vi "PS-RA03B FPGA.vi"() -> ()   [LabVIEW 2011]
uses:
  <vilib>/rvi/eio/common/nirviEmuTemplateMethod_errors.vi
  <vilib>/rvi/Memory/Memory_Emulation/niFpgaMemoryEmulationValidateCache.vi
  <vilib>/rvi/DataTransferAndStorage/Container/Common/niFpgaContainerGetUniqueNameForEmu.vi
  <vilib>/rvi/Memory/Memory_Emulation/nirvimemoryEmulationManagerCache_InsertValue.vi
  <vilib>/Utility/error.llb/Clear Errors.vi
  <vilib>/rvi/Memory/Memory_Emulation/nirvimemoryEmulationManagerCache_GetValue.vi
  <vilib>/rvi/Memory/Memory_Emulation/nirvimemoryEmulationManagerCache_SetValue.vi
  <vilib>/eio/EIONode/EIONode.xnode
  <vilib>/eio/EIOMethodNode/EIOMethodNode.xnode
  <vilib>/rvi/DataTransferAndStorage/Container/XNode/niFpgaContainer.xnode
  <vilib>/rvi/Memory/Memory_Emulation/nirvimemoryEmulation.vi
panel:
  out "Mod6/AO1":fxp<+/-,20,5> format="%.17g"
  out "Mod2/AO3":fxp<+/-,20,5> format="%.17g"
  out "Mod2/AO2":fxp<+/-,20,5> format="%.17g"
  out "Mod2/AO1":fxp<+/-,20,5> format="%.17g"
  out "Mod2/AO0":fxp<+/-,20,5> format="%.17g"
  out "Mod6/AO3":fxp<+/-,20,5> format="%.17g"
  out "Mod6/AO2":fxp<+/-,20,5> format="%.17g"
  out "Mod6/AO0":fxp<+/-,20,5> format="%.17g"
  out "Timestamp":u32 caption="Tick Count(Ticks)"
  out "Mod5/AI0":fxp<+/-,20,5> format="%.17g"
  out "Mod5/AI2":fxp<+/-,20,5> format="%.17g"
  out "Mod5/AI3":fxp<+/-,20,5> format="%.17g"
  out "Mod1/AI0":fxp<+/-,20,5> format="%.17g"
  out "Mod1/AI1":fxp<+/-,20,5> format="%.17g"
  out "Mod1/AI2":fxp<+/-,20,5> format="%.17g"
  out "Mod1/AI3":fxp<+/-,20,5> format="%.17g"
  out "Mod5/AI1":fxp<+/-,20,5> format="%.17g"
  out "period":u32
  out "delay":u32
  out "dperiod":u32
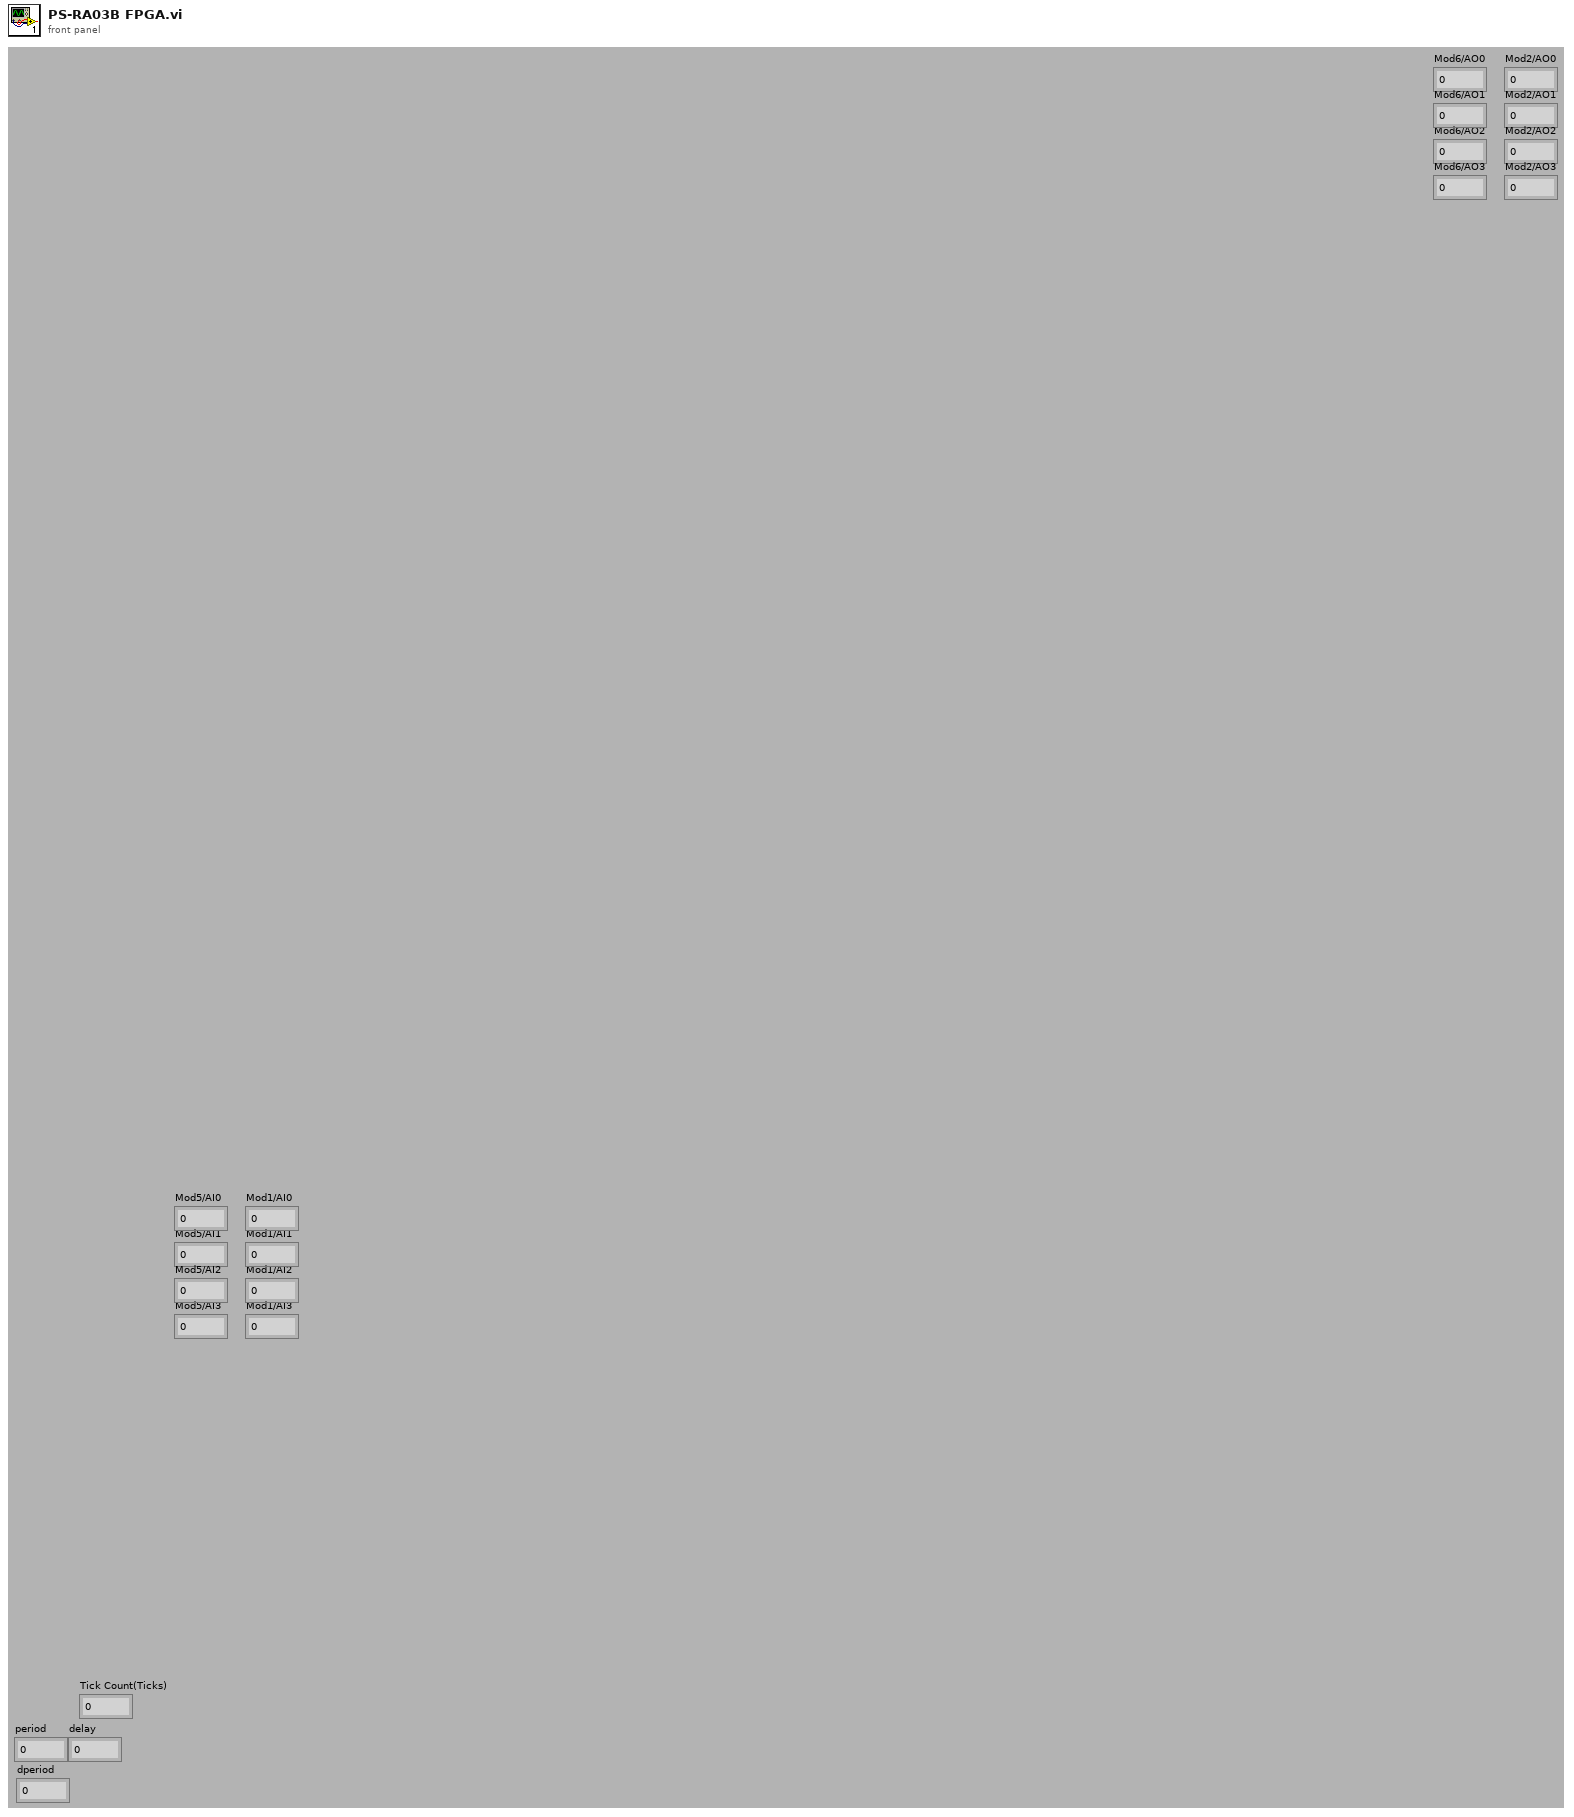
[diagram p1: front panel]
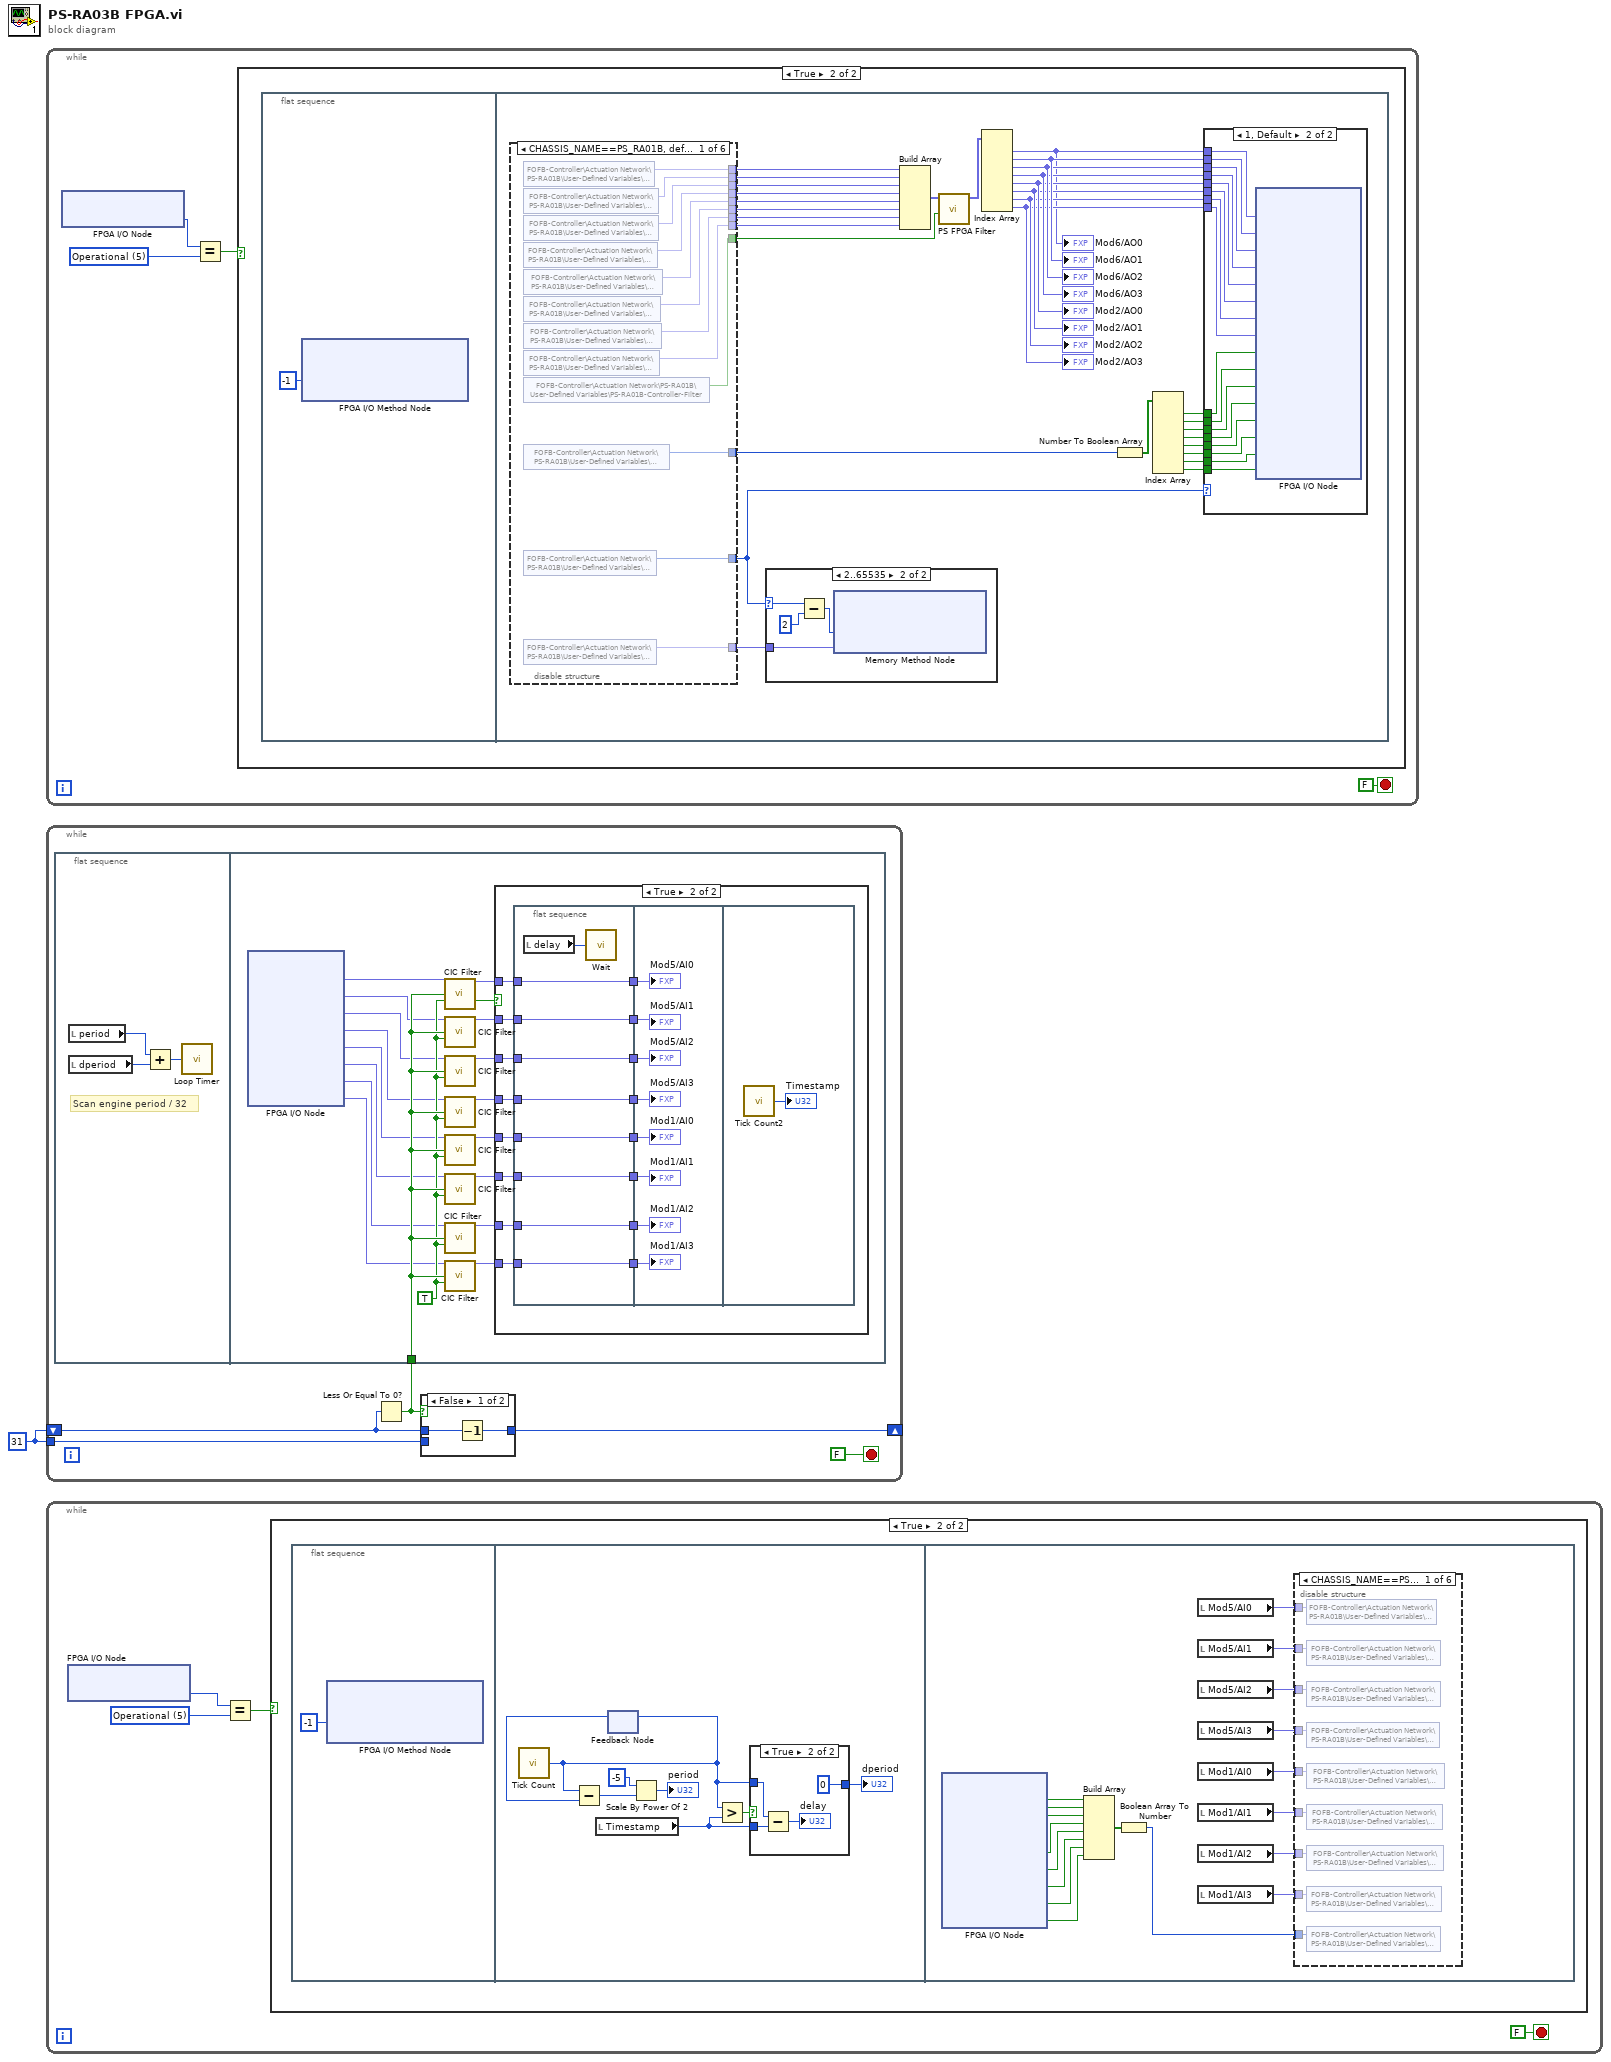
[diagram p0: block diagram]
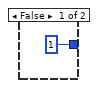
[diagram p5: hidden frame]
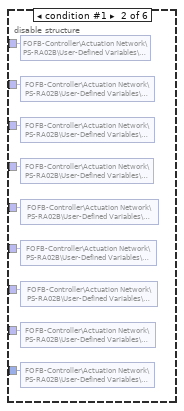
[diagram p6: hidden frame]
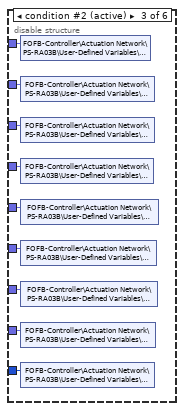
[diagram p7: hidden frame]
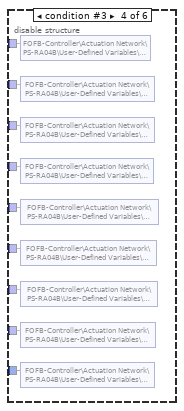
[diagram p8: hidden frame]
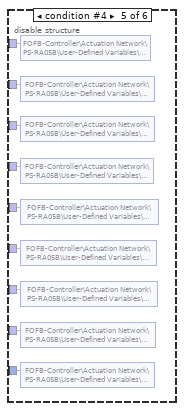
[diagram p9: hidden frame]
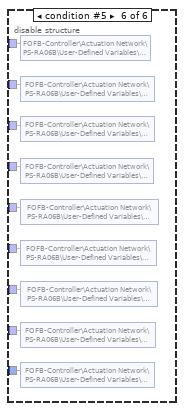
[diagram p10: hidden frame]
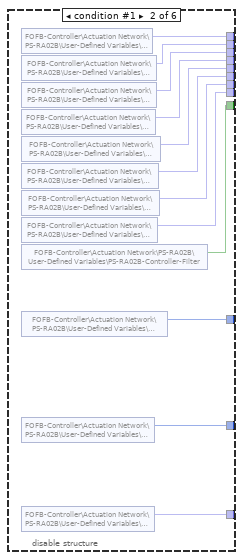
[diagram p14: hidden frame]
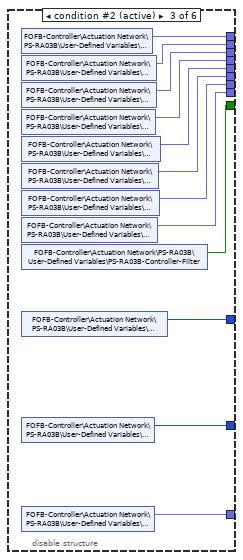
[diagram p15: hidden frame]
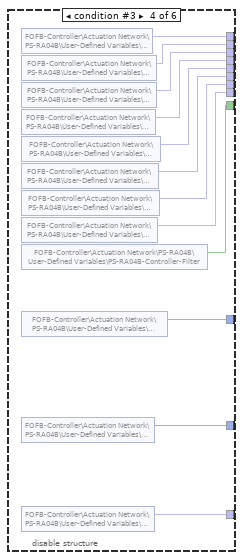
[diagram p16: hidden frame]
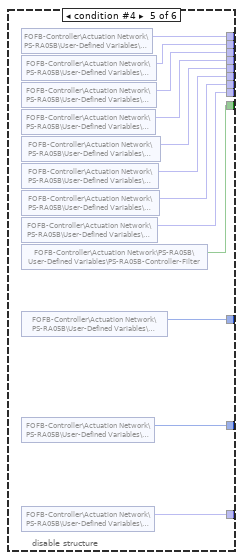
[diagram p17: hidden frame]
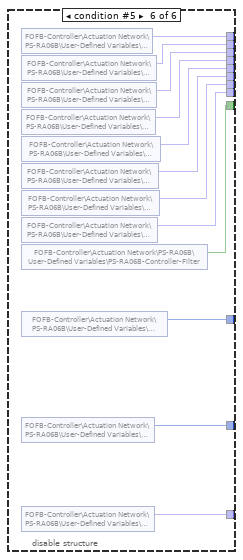
[diagram p18: hidden frame]
diagram:
  w1 = 31
  n1 = while {
    stop <- FALSE stop-if-true
    w2 = u8 5 items=["Init"=1, "PreOp"=2, "Bootstrap"=3, "SafeOp"=4, "Operational"=5]
    n2 = xnode "FPGA I/O Node"() -> ("EtherCAT State"=w3:u8)  [unwired: 1 in, 1 out]
    n3 = Equal?(x=w3, y=w2) -> (x = y?=w4:bool)
    n4 = case shown="True" w4 {
      frame False {
      }
      frame True {
        n5 = flat-sequence {
          frame #0 {
            n6 = xnode "FPGA I/O Method Node"("Timeout"=-1) -> ()  [unwired: 1 in, 2 out]
          }
          frame #1 {
            n7 = disable-structure shown="CHASSIS_NAME==PS_RA01B, default" {
              disable-tunnel: [w69 w70 w83 w101 w113 w129] -> w37
              disable-tunnel: [w68 w71 w84 w100 w112 w124] -> w36
              disable-tunnel: [w67 w72 w85 w99 w111 w123] -> w35
              disable-tunnel: [w66 w73 w86 w98 w110 w122] -> w34
              disable-tunnel: [w65 w74 w87 w97 w109 w121] -> w33
              disable-tunnel: [w64 w75 w88 w96 w108 w120] -> w32
              disable-tunnel: [w63 w76 w89 w95 w107 w119] -> w31
              disable-tunnel: [w62 w77 w90 w94 w106 w118] -> w30
              disable-tunnel: [w61 w81 w93 w105 w117 w128] -> w27
              disable-tunnel: [w60 w80 w92 w104 w116 w127] -> w29
              disable-tunnel: [w59 w79 w91 w103 w115 w126] -> w28
              disable-tunnel: [w58 w78 w82 w102 w114 w125] -> w7
              frame condition #0 {
                n8 = shared-variable "FOFB-Controller\\Actuation Network\\PS-RA01B\\User-Defined Variables\\ACH02-Setpoint"() -> (w69:fxp<+/-,20,5>)  [unwired: 1 in, 1 out]
                n9 = shared-variable "FOFB-Controller\\Actuation Network\\PS-RA01B\\User-Defined Variables\\RRA01B-Setpoint"() -> (w68:fxp<+/-,20,5>)  [unwired: 1 in, 1 out]
                n10 = shared-variable "FOFB-Controller\\Actuation Network\\PS-RA01B\\User-Defined Variables\\ALV02A-Setpoint"() -> (w67:fxp<+/-,20,5>)  [unwired: 1 in, 1 out]
                n11 = shared-variable "FOFB-Controller\\Actuation Network\\PS-RA01B\\User-Defined Variables\\ALV02B-Setpoint"() -> (w66:fxp<+/-,20,5>)  [unwired: 1 in, 1 out]
                n12 = shared-variable "FOFB-Controller\\Actuation Network\\PS-RA01B\\User-Defined Variables\\ACH03A-Setpoint"() -> (w65:fxp<+/-,20,5>)  [unwired: 1 in, 1 out]
                n13 = shared-variable "FOFB-Controller\\Actuation Network\\PS-RA01B\\User-Defined Variables\\ACV03A-Setpoint"() -> (w64:fxp<+/-,20,5>)  [unwired: 1 in, 1 out]
                n14 = shared-variable "FOFB-Controller\\Actuation Network\\PS-RA01B\\User-Defined Variables\\ACH01B-Setpoint"() -> (w63:fxp<+/-,20,5>)  [unwired: 1 in, 1 out]
                n15 = shared-variable "FOFB-Controller\\Actuation Network\\PS-RA01B\\User-Defined Variables\\ACV01B-Setpoint"() -> (w62:fxp<+/-,20,5>)  [unwired: 1 in, 1 out]
                n16 = shared-variable "FOFB-Controller\\Actuation Network\\PS-RA01B\\User-Defined Variables\\PS-RA01B-Controller-Filter"() -> (w60:bool)  [unwired: 1 in, 1 out]
                n17 = shared-variable "FOFB-Controller\\Actuation Network\\PS-RA01B\\User-Defined Variables\\PS-RA01B-ON-OFF"() -> (w61:u8)  [unwired: 1 in, 1 out]
                n18 = shared-variable "FOFB-Controller\\Actuation Network\\PS-RA01B\\User-Defined Variables\\PS-RA01B-ADDR"() -> (w58:u16)  [unwired: 1 in, 1 out]
                n19 = shared-variable "FOFB-Controller\\Actuation Network\\PS-RA01B\\User-Defined Variables\\PS-RA01B-DATA"() -> (w59:fxp<+/-,22,4>)  [unwired: 1 in, 1 out]
              }
              frame condition #1 {
                n20 = shared-variable "FOFB-Controller\\Actuation Network\\PS-RA02B\\User-Defined Variables\\ACH04-Setpoint"() -> (w70:fxp<+/-,20,5>)  [unwired: 1 in, 1 out]
                n21 = shared-variable "FOFB-Controller\\Actuation Network\\PS-RA02B\\User-Defined Variables\\RRA02B-Setpoint"() -> (w71:fxp<+/-,20,5>)  [unwired: 1 in, 1 out]
                n22 = shared-variable "FOFB-Controller\\Actuation Network\\PS-RA02B\\User-Defined Variables\\ALV04A-Setpoint"() -> (w72:fxp<+/-,20,5>)  [unwired: 1 in, 1 out]
                n23 = shared-variable "FOFB-Controller\\Actuation Network\\PS-RA02B\\User-Defined Variables\\ALV04B-Setpoint"() -> (w73:fxp<+/-,20,5>)  [unwired: 1 in, 1 out]
                n24 = shared-variable "FOFB-Controller\\Actuation Network\\PS-RA02B\\User-Defined Variables\\ACH05A-Setpoint"() -> (w74:fxp<+/-,20,5>)  [unwired: 1 in, 1 out]
                n25 = shared-variable "FOFB-Controller\\Actuation Network\\PS-RA02B\\User-Defined Variables\\ACV05A-Setpoint"() -> (w75:fxp<+/-,20,5>)  [unwired: 1 in, 1 out]
                n26 = shared-variable "FOFB-Controller\\Actuation Network\\PS-RA02B\\User-Defined Variables\\ACH03B-Setpoint"() -> (w76:fxp<+/-,20,5>)  [unwired: 1 in, 1 out]
                n27 = shared-variable "FOFB-Controller\\Actuation Network\\PS-RA02B\\User-Defined Variables\\ACV03B-Setpoint"() -> (w77:fxp<+/-,20,5>)  [unwired: 1 in, 1 out]
                n28 = shared-variable "FOFB-Controller\\Actuation Network\\PS-RA02B\\User-Defined Variables\\PS-RA02B-Controller-Filter"() -> (w80:bool)  [unwired: 1 in, 1 out]
                n29 = shared-variable "FOFB-Controller\\Actuation Network\\PS-RA02B\\User-Defined Variables\\PS-RA02B-ON-OFF"() -> (w81:u8)  [unwired: 1 in, 1 out]
                n30 = shared-variable "FOFB-Controller\\Actuation Network\\PS-RA02B\\User-Defined Variables\\PS-RA02B-ADDR"() -> (w78:u16)  [unwired: 1 in, 1 out]
                n31 = shared-variable "FOFB-Controller\\Actuation Network\\PS-RA02B\\User-Defined Variables\\PS-RA02B-DATA"() -> (w79:fxp<+/-,22,4>)  [unwired: 1 in, 1 out]
              }
              frame condition #2 (active) {
                n32 = shared-variable "FOFB-Controller\\Actuation Network\\PS-RA03B\\User-Defined Variables\\ACH06-Setpoint"() -> (w83:fxp<+/-,20,5>)  [unwired: 1 in, 1 out]
                n33 = shared-variable "FOFB-Controller\\Actuation Network\\PS-RA03B\\User-Defined Variables\\RRA03B-Setpoint"() -> (w84:fxp<+/-,20,5>)  [unwired: 1 in, 1 out]
                n34 = shared-variable "FOFB-Controller\\Actuation Network\\PS-RA03B\\User-Defined Variables\\ALV06A-Setpoint"() -> (w85:fxp<+/-,20,5>)  [unwired: 1 in, 1 out]
                n35 = shared-variable "FOFB-Controller\\Actuation Network\\PS-RA03B\\User-Defined Variables\\ALV06B-Setpoint"() -> (w86:fxp<+/-,20,5>)  [unwired: 1 in, 1 out]
                n36 = shared-variable "FOFB-Controller\\Actuation Network\\PS-RA03B\\User-Defined Variables\\ACH07A-Setpoint"() -> (w87:fxp<+/-,20,5>)  [unwired: 1 in, 1 out]
                n37 = shared-variable "FOFB-Controller\\Actuation Network\\PS-RA03B\\User-Defined Variables\\ACV07A-Setpoint"() -> (w88:fxp<+/-,20,5>)  [unwired: 1 in, 1 out]
                n38 = shared-variable "FOFB-Controller\\Actuation Network\\PS-RA03B\\User-Defined Variables\\ACH05B-Setpoint"() -> (w89:fxp<+/-,20,5>)  [unwired: 1 in, 1 out]
                n39 = shared-variable "FOFB-Controller\\Actuation Network\\PS-RA03B\\User-Defined Variables\\ACV05B-Setpoint"() -> (w90:fxp<+/-,20,5>)  [unwired: 1 in, 1 out]
                n40 = shared-variable "FOFB-Controller\\Actuation Network\\PS-RA03B\\User-Defined Variables\\PS-RA03B-Controller-Filter"() -> (w92:bool)  [unwired: 1 in, 1 out]
                n41 = shared-variable "FOFB-Controller\\Actuation Network\\PS-RA03B\\User-Defined Variables\\PS-RA03B-ON-OFF"() -> (w93:u8)  [unwired: 1 in, 1 out]
                n42 = shared-variable "FOFB-Controller\\Actuation Network\\PS-RA03B\\User-Defined Variables\\PS-RA03B-ADDR"() -> (w82:u16)  [unwired: 1 in, 1 out]
                n43 = shared-variable "FOFB-Controller\\Actuation Network\\PS-RA03B\\User-Defined Variables\\PS-RA03B-DATA"() -> (w91:fxp<+/-,22,4>)  [unwired: 1 in, 1 out]
              }
              frame condition #3 {
                n44 = shared-variable "FOFB-Controller\\Actuation Network\\PS-RA04B\\User-Defined Variables\\ACH08-Setpoint"() -> (w101:fxp<+/-,20,5>)  [unwired: 1 in, 1 out]
                n45 = shared-variable "FOFB-Controller\\Actuation Network\\PS-RA04B\\User-Defined Variables\\RRA04B-Setpoint"() -> (w100:fxp<+/-,20,5>)  [unwired: 1 in, 1 out]
                n46 = shared-variable "FOFB-Controller\\Actuation Network\\PS-RA04B\\User-Defined Variables\\ALV08A-Setpoint"() -> (w99:fxp<+/-,20,5>)  [unwired: 1 in, 1 out]
                n47 = shared-variable "FOFB-Controller\\Actuation Network\\PS-RA04B\\User-Defined Variables\\ALV08B-Setpoint"() -> (w98:fxp<+/-,20,5>)  [unwired: 1 in, 1 out]
                n48 = shared-variable "FOFB-Controller\\Actuation Network\\PS-RA04B\\User-Defined Variables\\ACH09A-Setpoint"() -> (w97:fxp<+/-,20,5>)  [unwired: 1 in, 1 out]
                n49 = shared-variable "FOFB-Controller\\Actuation Network\\PS-RA04B\\User-Defined Variables\\ACV09A-Setpoint"() -> (w96:fxp<+/-,20,5>)  [unwired: 1 in, 1 out]
                n50 = shared-variable "FOFB-Controller\\Actuation Network\\PS-RA04B\\User-Defined Variables\\ACH07B-Setpoint"() -> (w95:fxp<+/-,20,5>)  [unwired: 1 in, 1 out]
                n51 = shared-variable "FOFB-Controller\\Actuation Network\\PS-RA04B\\User-Defined Variables\\ACV07B-Setpoint"() -> (w94:fxp<+/-,20,5>)  [unwired: 1 in, 1 out]
                n52 = shared-variable "FOFB-Controller\\Actuation Network\\PS-RA04B\\User-Defined Variables\\PS-RA04B-Controller-Filter"() -> (w104:bool)  [unwired: 1 in, 1 out]
                n53 = shared-variable "FOFB-Controller\\Actuation Network\\PS-RA04B\\User-Defined Variables\\PS-RA04B-ON-OFF"() -> (w105:u8)  [unwired: 1 in, 1 out]
                n54 = shared-variable "FOFB-Controller\\Actuation Network\\PS-RA04B\\User-Defined Variables\\PS-RA04B-ADDR"() -> (w102:u16)  [unwired: 1 in, 1 out]
                n55 = shared-variable "FOFB-Controller\\Actuation Network\\PS-RA04B\\User-Defined Variables\\PS-RA04B-DATA"() -> (w103:fxp<+/-,22,4>)  [unwired: 1 in, 1 out]
              }
              frame condition #4 {
                n56 = shared-variable "FOFB-Controller\\Actuation Network\\PS-RA05B\\User-Defined Variables\\ACH10-Setpoint"() -> (w113:fxp<+/-,20,5>)  [unwired: 1 in, 1 out]
                n57 = shared-variable "FOFB-Controller\\Actuation Network\\PS-RA05B\\User-Defined Variables\\RRA05B-Setpoint"() -> (w112:fxp<+/-,20,5>)  [unwired: 1 in, 1 out]
                n58 = shared-variable "FOFB-Controller\\Actuation Network\\PS-RA05B\\User-Defined Variables\\ALV10A-Setpoint"() -> (w111:fxp<+/-,20,5>)  [unwired: 1 in, 1 out]
                n59 = shared-variable "FOFB-Controller\\Actuation Network\\PS-RA05B\\User-Defined Variables\\ALV10B-Setpoint"() -> (w110:fxp<+/-,20,5>)  [unwired: 1 in, 1 out]
                n60 = shared-variable "FOFB-Controller\\Actuation Network\\PS-RA05B\\User-Defined Variables\\ACH11A-Setpoint"() -> (w109:fxp<+/-,20,5>)  [unwired: 1 in, 1 out]
                n61 = shared-variable "FOFB-Controller\\Actuation Network\\PS-RA05B\\User-Defined Variables\\ACV11A-Setpoint"() -> (w108:fxp<+/-,20,5>)  [unwired: 1 in, 1 out]
                n62 = shared-variable "FOFB-Controller\\Actuation Network\\PS-RA05B\\User-Defined Variables\\ACH09B-Setpoint"() -> (w107:fxp<+/-,20,5>)  [unwired: 1 in, 1 out]
                n63 = shared-variable "FOFB-Controller\\Actuation Network\\PS-RA05B\\User-Defined Variables\\ACV09B-Setpoint"() -> (w106:fxp<+/-,20,5>)  [unwired: 1 in, 1 out]
                n64 = shared-variable "FOFB-Controller\\Actuation Network\\PS-RA05B\\User-Defined Variables\\PS-RA05B-Controller-Filter"() -> (w116:bool)  [unwired: 1 in, 1 out]
                n65 = shared-variable "FOFB-Controller\\Actuation Network\\PS-RA05B\\User-Defined Variables\\PS-RA05B-ON-OFF"() -> (w117:u8)  [unwired: 1 in, 1 out]
                n66 = shared-variable "FOFB-Controller\\Actuation Network\\PS-RA05B\\User-Defined Variables\\PS-RA05B-ADDR"() -> (w114:u16)  [unwired: 1 in, 1 out]
                n67 = shared-variable "FOFB-Controller\\Actuation Network\\PS-RA05B\\User-Defined Variables\\PS-RA05B-DATA"() -> (w115:fxp<+/-,22,4>)  [unwired: 1 in, 1 out]
              }
              frame condition #5 {
                n68 = shared-variable "FOFB-Controller\\Actuation Network\\PS-RA06B\\User-Defined Variables\\ACH12-Setpoint"() -> (w129:fxp<+/-,20,5>)  [unwired: 1 in, 1 out]
                n69 = shared-variable "FOFB-Controller\\Actuation Network\\PS-RA06B\\User-Defined Variables\\RRA06B-Setpoint"() -> (w124:fxp<+/-,20,5>)  [unwired: 1 in, 1 out]
                n70 = shared-variable "FOFB-Controller\\Actuation Network\\PS-RA06B\\User-Defined Variables\\ALV12A-Setpoint"() -> (w123:fxp<+/-,20,5>)  [unwired: 1 in, 1 out]
                n71 = shared-variable "FOFB-Controller\\Actuation Network\\PS-RA06B\\User-Defined Variables\\ALV12B-Setpoint"() -> (w122:fxp<+/-,20,5>)  [unwired: 1 in, 1 out]
                n72 = shared-variable "FOFB-Controller\\Actuation Network\\PS-RA06B\\User-Defined Variables\\ACH01A-Setpoint"() -> (w121:fxp<+/-,20,5>)  [unwired: 1 in, 1 out]
                n73 = shared-variable "FOFB-Controller\\Actuation Network\\PS-RA06B\\User-Defined Variables\\ACV01A-Setpoint"() -> (w120:fxp<+/-,20,5>)  [unwired: 1 in, 1 out]
                n74 = shared-variable "FOFB-Controller\\Actuation Network\\PS-RA06B\\User-Defined Variables\\ACH11B-Setpoint"() -> (w119:fxp<+/-,20,5>)  [unwired: 1 in, 1 out]
                n75 = shared-variable "FOFB-Controller\\Actuation Network\\PS-RA06B\\User-Defined Variables\\ACV11B-Setpoint"() -> (w118:fxp<+/-,20,5>)  [unwired: 1 in, 1 out]
                n76 = shared-variable "FOFB-Controller\\Actuation Network\\PS-RA06B\\User-Defined Variables\\PS-RA06B-Controller-Filter"() -> (w127:bool)  [unwired: 1 in, 1 out]
                n77 = shared-variable "FOFB-Controller\\Actuation Network\\PS-RA06B\\User-Defined Variables\\PS-RA06B-ON-OFF"() -> (w128:u8)  [unwired: 1 in, 1 out]
                n78 = shared-variable "FOFB-Controller\\Actuation Network\\PS-RA06B\\User-Defined Variables\\PS-RA06B-ADDR"() -> (w125:u16)  [unwired: 1 in, 1 out]
                n79 = shared-variable "FOFB-Controller\\Actuation Network\\PS-RA06B\\User-Defined Variables\\PS-RA06B-DATA"() -> (w126:fxp<+/-,22,4>)  [unwired: 1 in, 1 out]
              }
            }
            n80 = case shown="2..65535" w7 {
              selector: w7 -> [_ w57]
              tunnel: w28 -> [_ w54]
              frame 0, Default {
              }
              frame 2..65535 {
                n81 = Subtract(x=w57, y=u16 2) -> (x-y=w55:u16)
                n82 = xnode ("Memory Method Node")("Address"=w55, "Data"=w54) -> ()  [unwired: 1 in, 1 out]
              }
            }
            n83 = Build Array(w37, w36, w35, w34, w33, w32, w31, w30) -> (w26:fxp<+/-,20,5>[])
            n84 = call "PS FPGA Filter.vi"("filter?"=w29, "input"=w26) -> ("output"=w25:fxp<+/-,20,5>[])  [unwired: 8 in, 1 out]
            n85 = Index Array(array=w25) -> (element #1=w8:fxp<+/-,20,5>, element #2=w24:fxp<+/-,20,5>, element #3=w23:fxp<+/-,20,5>, element #4=w22:fxp<+/-,20,5>, element #5=w21:fxp<+/-,20,5>, element #6=w20:fxp<+/-,20,5>, element #7=w19:fxp<+/-,20,5>, element #8=w18:fxp<+/-,20,5>)  [unwired: 8 in]
            "Mod6/AO0" <- w8
            "Mod6/AO2" <- w23
            "Mod6/AO3" <- w22
            "Mod2/AO0" <- w21
            "Mod2/AO1" <- w20
            "Mod2/AO2" <- w19
            "Mod2/AO3" <- w18
            "Mod6/AO1" <- w24
            n86 = Number To Boolean Array(number=w27) -> (Boolean array=w17:bool[])
            n87 = Index Array(array=w17) -> (element #1=w16:bool, element #2=w15:bool, element #3=w14:bool, element #4=w13:bool, element #5=w12:bool, element #6=w9:bool, element #7=w10:bool, element #8=w11:bool)  [unwired: 8 in]
            n88 = case shown="1, Default" w7 {
              tunnel: w24 -> [_ w53]
              tunnel: w23 -> [_ w52]
              tunnel: w22 -> [_ w51]
              tunnel: w21 -> [_ w50]
              tunnel: w20 -> [_ w49]
              tunnel: w19 -> [_ w48]
              tunnel: w18 -> [_ w47]
              tunnel: w16 -> [_ w46]
              tunnel: w15 -> [_ w45]
              tunnel: w14 -> [_ w44]
              tunnel: w13 -> [_ w43]
              tunnel: w12 -> [_ w42]
              tunnel: w11 -> [_ w41]
              tunnel: w10 -> [_ w40]
              tunnel: w9 -> [_ w39]
              tunnel: w8 -> [_ w38]
              frame 0 {
              }
              frame 1, Default {
                n89 = xnode "FPGA I/O Node"("Mod6/AO0"=w38, "Mod6/AO1"=w53, "Mod6/AO2"=w52, "Mod6/AO3"=w51, "Mod2/AO0"=w50, "Mod2/AO1"=w49, "Mod2/AO2"=w48, "Mod2/AO3"=w47, "Mod4/DIO6"=w46, "Mod4/DIO7"=w45, "Mod4/DIO4"=w44, "Mod4/DIO5"=w43, "Mod4/DIO2"=w42, "Mod4/DIO3"=w39, "Mod4/DIO0"=w40, "Mod4/DIO1"=w41) -> ()  [unwired: 16 in, 16 out]
              }
            }
          }
        }
      }
    }
  }
  n90 = while {
    shift-right: [w133] -> _
    shift-left: w1 -> [w132]
    tunnel: w1 -> [w130]
    stop <- FALSE stop-if-true
    n91 = flat-sequence {
      tunnel: w131 -> [w159]
      frame #0 {
        # "Scan engine period / 32"
        n92 = local read "period"() -> (w140:u32)
        n93 = local read "dperiod"() -> (w139:u32)
        n94 = Add(x=w140, y=w139) -> (x+y=w138:u32)
        n95 = call "Loop Timer"("Count(Ticks)"=w138) -> ()  [unwired: 1 out]
      }
      frame #1 {
        w158 = TRUE ("input valid")
        n96 = xnode "FPGA I/O Node"() -> ("Mod5/AI0"=w157:fxp<+/-,20,5>, "Mod5/AI1"=w156:fxp<+/-,20,5>, "Mod5/AI2"=w155:fxp<+/-,20,5>, "Mod5/AI3"=w154:fxp<+/-,20,5>, "Mod1/AI0"=w153:fxp<+/-,20,5>, "Mod1/AI1"=w152:fxp<+/-,20,5>, "Mod1/AI2"=w151:fxp<+/-,20,5>, "Mod1/AI3"=w150:fxp<+/-,20,5>)  [unwired: 8 in, 8 out]
        n97 = call "CIC Filter.vi"("input data"=w157, "sample"=w159, "input valid"=w158) -> ("output data"=w148:fxp<+/-,20,5>, "output valid"=w149:bool)  [unwired: 10 in, 1 out]
        n98 = call "CIC Filter.vi"("input data"=w156, "sample"=w159, "input valid"=w158) -> ("output data"=w147:fxp<+/-,20,5>)  [unwired: 10 in, 2 out]
        n99 = call "CIC Filter.vi"("input data"=w155, "sample"=w159, "input valid"=w158) -> ("output data"=w146:fxp<+/-,20,5>)  [unwired: 10 in, 2 out]
        n100 = call "CIC Filter.vi"("input data"=w154, "sample"=w159, "input valid"=w158) -> ("output data"=w145:fxp<+/-,20,5>)  [unwired: 10 in, 2 out]
        n101 = call "CIC Filter.vi"("input data"=w153, "sample"=w159, "input valid"=w158) -> ("output data"=w144:fxp<+/-,20,5>)  [unwired: 10 in, 2 out]
        n102 = call "CIC Filter.vi"("input data"=w152, "sample"=w159, "input valid"=w158) -> ("output data"=w143:fxp<+/-,20,5>)  [unwired: 10 in, 2 out]
        n103 = call "CIC Filter.vi"("input data"=w151, "sample"=w159, "input valid"=w158) -> ("output data"=w142:fxp<+/-,20,5>)  [unwired: 10 in, 2 out]
        n104 = call "CIC Filter.vi"("input data"=w150, "sample"=w159, "input valid"=w158) -> ("output data"=w141:fxp<+/-,20,5>)  [unwired: 10 in, 2 out]
        n105 = case shown="True" w149 {
          tunnel: w148 -> [_ w175]
          tunnel: w147 -> [_ w173]
          tunnel: w146 -> [_ w171]
          tunnel: w145 -> [_ w170]
          tunnel: w144 -> [_ w167]
          tunnel: w143 -> [_ w165]
          tunnel: w142 -> [_ w163]
          tunnel: w141 -> [_ w161]
          frame False {
          }
          frame True {
            n106 = flat-sequence {
              tunnel: w175 -> [w184]
              tunnel: [w184] -> w174
              tunnel: w173 -> [w182]
              tunnel: [w182] -> w172
              tunnel: w171 -> [w180]
              tunnel: w170 -> [w181]
              tunnel: [w181] -> w169
              tunnel: [w180] -> w168
              tunnel: w167 -> [w179]
              tunnel: [w179] -> w166
              tunnel: w165 -> [w178]
              tunnel: [w178] -> w164
              tunnel: w163 -> [w177]
              tunnel: [w177] -> w162
              tunnel: w161 -> [w176]
              tunnel: [w176] -> w160
              tunnel: w174 -> [w191]
              tunnel: w172 -> [w192]
              tunnel: w169 -> [w190]
              tunnel: w168 -> [w189]
              tunnel: w166 -> [w188]
              tunnel: w164 -> [w187]
              tunnel: w162 -> [w186]
              tunnel: w160 -> [w185]
              frame #0 {
                n107 = local read "delay"() -> (w183:u32)
                n108 = call "Wait"("Count(Ticks)"=w183) -> ()  [unwired: 1 out]
              }
              frame #1 {
                "Mod5/AI0" <- w191
                "Mod5/AI2" <- w189
                "Mod5/AI3" <- w190
                "Mod1/AI0" <- w188
                "Mod1/AI1" <- w187
                "Mod1/AI2" <- w186
                "Mod1/AI3" <- w185
                "Mod5/AI1" <- w192
              }
              frame #2 {
                n109 = call "Tick Count2"() -> ("Tick Count(Ticks)"=→"Timestamp":u32)
              }
            }
          }
        }
      }
    }
    n110 = Less Or Equal To 0?(x=w132) -> (x <= 0?=w131:bool)
    n111 = case shown="False" w131 {
      tunnel: [w136 w137] -> w133
      tunnel: w132 -> [w135 _]
      tunnel: w130 -> [_ w137]
      frame False {
        n112 = Decrement(x=w135) -> (x-1=w136:i32)
      }
      frame True {
      }
    }
  }
  n113 = while {
    stop <- FALSE stop-if-true
    w196 = u8 5 items=["Init"=1, "PreOp"=2, "Bootstrap"=3, "SafeOp"=4, "Operational"=5]
    n114 = xnode "FPGA I/O Node"() -> ("EtherCAT State"=w195:u8)  [unwired: 1 in, 1 out]
    n115 = Equal?(x=w195, y=w196) -> (x = y?=w194:bool)
    n116 = case shown="True" w194 {
      frame False {
      }
      frame True {
        n117 = flat-sequence {
          frame #0 {
            n118 = xnode "FPGA I/O Method Node"("Timeout"=-1) -> ()  [unwired: 1 in, 2 out]
          }
          frame #1 {
            n119 = call "Tick Count"() -> ("Tick Count(Ticks)"=w200:u32)
            n120 = local read "Timestamp"() -> (w202:u32)
            n121 = feedback #1() -> (w199:u32)  [unwired: 1 in]
            n122 = Subtract(x=w200, y=w199) -> (x-y=w205:u32)
            n123 = feedback-in #1(w200) -> ()
            n124 = Scale By Power Of 2(n=i8 -5, x=w205) -> (x*2^n=→"period":u32)
            n125 = Greater?(x=w200, y=w202) -> (0:w203:bool)
            n126 = case shown="True" w203 {
              tunnel: w200 -> [_ w211]
              tunnel: w202 -> [_ w210]
              tunnel: [u32 1 ("dt 2") u32 0 ("dt 2")] -> w201
              frame False {
              }
              frame True {
                n127 = Subtract(x=w211, y=w210) -> (x-y=→"delay":u32)
              }
            }
            "dperiod" <- w201
          }
          frame #2 {
            n128 = xnode "FPGA I/O Node"() -> ("Mod3/DIO6"=w214:bool, "Mod3/DIO7"=w215:bool, "Mod3/DIO4"=w216:bool, "Mod3/DIO5"=w217:bool, "Mod3/DIO2"=w218:bool, "Mod3/DIO3"=w219:bool, "Mod3/DIO0"=w220:bool, "Mod3/DIO1"=w221:bool)  [unwired: 8 in, 8 out]
            n129 = Build Array(w214, w215, w216, w217, w218, w219, w220, w221) -> (w213:bool[])
            n130 = Boolean Array To Number(Boolean array=w213) -> (number=w212:u8)
            n131 = local read "Mod5/AI0"() -> (w229:fxp<+/-,20,5>)
            n132 = local read "Mod5/AI1"() -> (w228:fxp<+/-,20,5>)
            n133 = local read "Mod5/AI2"() -> (w227:fxp<+/-,20,5>)
            n134 = local read "Mod5/AI3"() -> (w226:fxp<+/-,20,5>)
            n135 = local read "Mod1/AI0"() -> (w225:fxp<+/-,20,5>)
            n136 = local read "Mod1/AI1"() -> (w224:fxp<+/-,20,5>)
            n137 = local read "Mod1/AI2"() -> (w223:fxp<+/-,20,5>)
            n138 = local read "Mod1/AI3"() -> (w222:fxp<+/-,20,5>)
            n139 = disable-structure shown="CHASSIS_NAME==PS_RA01B, default" {
              disable-tunnel: w229 -> [w238 w246 w255 w264 w273 w282]
              disable-tunnel: w228 -> [w237 w245 w254 w263 w272 w281]
              disable-tunnel: w227 -> [w236 w244 w253 w262 w271 w280]
              disable-tunnel: w226 -> [w235 w243 w252 w261 w270 w279]
              disable-tunnel: w225 -> [w234 w242 w251 w260 w269 w278]
              disable-tunnel: w224 -> [w233 w241 w250 w259 w268 w277]
              disable-tunnel: w223 -> [w232 w240 w249 w258 w267 w276]
              disable-tunnel: w222 -> [w231 w239 w248 w257 w266 w275]
              disable-tunnel: w212 -> [w230 w247 w256 w265 w274 w283]
              frame condition #0 {
                n140 = shared-variable "FOFB-Controller\\Actuation Network\\PS-RA01B\\User-Defined Variables\\ACH02-Reading"(w238) -> ()  [unwired: 1 in, 1 out]
                n141 = shared-variable "FOFB-Controller\\Actuation Network\\PS-RA01B\\User-Defined Variables\\RRA01B-Reading"(w237) -> ()  [unwired: 1 in, 1 out]
                n142 = shared-variable "FOFB-Controller\\Actuation Network\\PS-RA01B\\User-Defined Variables\\ALV02A-Reading"(w236) -> ()  [unwired: 1 in, 1 out]
                n143 = shared-variable "FOFB-Controller\\Actuation Network\\PS-RA01B\\User-Defined Variables\\ALV02B-Reading"(w235) -> ()  [unwired: 1 in, 1 out]
                n144 = shared-variable "FOFB-Controller\\Actuation Network\\PS-RA01B\\User-Defined Variables\\ACH03A-Reading"(w234) -> ()  [unwired: 1 in, 1 out]
                n145 = shared-variable "FOFB-Controller\\Actuation Network\\PS-RA01B\\User-Defined Variables\\ACV03A-Reading"(w233) -> ()  [unwired: 1 in, 1 out]
                n146 = shared-variable "FOFB-Controller\\Actuation Network\\PS-RA01B\\User-Defined Variables\\ACH01B-Reading"(w232) -> ()  [unwired: 1 in, 1 out]
                n147 = shared-variable "FOFB-Controller\\Actuation Network\\PS-RA01B\\User-Defined Variables\\ACV01B-Reading"(w231) -> ()  [unwired: 1 in, 1 out]
                n148 = shared-variable "FOFB-Controller\\Actuation Network\\PS-RA01B\\User-Defined Variables\\PS-RA01B-Status"(w230) -> ()  [unwired: 1 in, 1 out]
              }
              frame condition #1 {
                n149 = shared-variable "FOFB-Controller\\Actuation Network\\PS-RA02B\\User-Defined Variables\\ACH04-Reading"(w246) -> ()  [unwired: 1 in, 1 out]
                n150 = shared-variable "FOFB-Controller\\Actuation Network\\PS-RA02B\\User-Defined Variables\\RRA02B-Reading"(w245) -> ()  [unwired: 1 in, 1 out]
                n151 = shared-variable "FOFB-Controller\\Actuation Network\\PS-RA02B\\User-Defined Variables\\ALV04A-Reading"(w244) -> ()  [unwired: 1 in, 1 out]
                n152 = shared-variable "FOFB-Controller\\Actuation Network\\PS-RA02B\\User-Defined Variables\\ALV04B-Reading"(w243) -> ()  [unwired: 1 in, 1 out]
                n153 = shared-variable "FOFB-Controller\\Actuation Network\\PS-RA02B\\User-Defined Variables\\ACH05A-Reading"(w242) -> ()  [unwired: 1 in, 1 out]
                n154 = shared-variable "FOFB-Controller\\Actuation Network\\PS-RA02B\\User-Defined Variables\\ACV05A-Reading"(w241) -> ()  [unwired: 1 in, 1 out]
                n155 = shared-variable "FOFB-Controller\\Actuation Network\\PS-RA02B\\User-Defined Variables\\ACH03B-Reading"(w240) -> ()  [unwired: 1 in, 1 out]
                n156 = shared-variable "FOFB-Controller\\Actuation Network\\PS-RA02B\\User-Defined Variables\\ACV03B-Reading"(w239) -> ()  [unwired: 1 in, 1 out]
                n157 = shared-variable "FOFB-Controller\\Actuation Network\\PS-RA02B\\User-Defined Variables\\PS-RA02B-Status"(w247) -> ()  [unwired: 1 in, 1 out]
              }
              frame condition #2 (active) {
                n158 = shared-variable "FOFB-Controller\\Actuation Network\\PS-RA03B\\User-Defined Variables\\ACH06-Reading"(w255) -> ()  [unwired: 1 in, 1 out]
                n159 = shared-variable "FOFB-Controller\\Actuation Network\\PS-RA03B\\User-Defined Variables\\RRA03B-Reading"(w254) -> ()  [unwired: 1 in, 1 out]
                n160 = shared-variable "FOFB-Controller\\Actuation Network\\PS-RA03B\\User-Defined Variables\\ALV06A-Reading"(w253) -> ()  [unwired: 1 in, 1 out]
                n161 = shared-variable "FOFB-Controller\\Actuation Network\\PS-RA03B\\User-Defined Variables\\ALV06B-Reading"(w252) -> ()  [unwired: 1 in, 1 out]
                n162 = shared-variable "FOFB-Controller\\Actuation Network\\PS-RA03B\\User-Defined Variables\\ACH07A-Reading"(w251) -> ()  [unwired: 1 in, 1 out]
                n163 = shared-variable "FOFB-Controller\\Actuation Network\\PS-RA03B\\User-Defined Variables\\ACV07A-Reading"(w250) -> ()  [unwired: 1 in, 1 out]
                n164 = shared-variable "FOFB-Controller\\Actuation Network\\PS-RA03B\\User-Defined Variables\\ACH05B-Reading"(w249) -> ()  [unwired: 1 in, 1 out]
                n165 = shared-variable "FOFB-Controller\\Actuation Network\\PS-RA03B\\User-Defined Variables\\ACV05B-Reading"(w248) -> ()  [unwired: 1 in, 1 out]
                n166 = shared-variable "FOFB-Controller\\Actuation Network\\PS-RA03B\\User-Defined Variables\\PS-RA03B-Status"(w256) -> ()  [unwired: 1 in, 1 out]
              }
              frame condition #3 {
                n167 = shared-variable "FOFB-Controller\\Actuation Network\\PS-RA04B\\User-Defined Variables\\ACH08-Reading"(w264) -> ()  [unwired: 1 in, 1 out]
                n168 = shared-variable "FOFB-Controller\\Actuation Network\\PS-RA04B\\User-Defined Variables\\RRA04B-Reading"(w263) -> ()  [unwired: 1 in, 1 out]
                n169 = shared-variable "FOFB-Controller\\Actuation Network\\PS-RA04B\\User-Defined Variables\\ALV08A-Reading"(w262) -> ()  [unwired: 1 in, 1 out]
                n170 = shared-variable "FOFB-Controller\\Actuation Network\\PS-RA04B\\User-Defined Variables\\ALV08B-Reading"(w261) -> ()  [unwired: 1 in, 1 out]
                n171 = shared-variable "FOFB-Controller\\Actuation Network\\PS-RA04B\\User-Defined Variables\\ACH09A-Reading"(w260) -> ()  [unwired: 1 in, 1 out]
                n172 = shared-variable "FOFB-Controller\\Actuation Network\\PS-RA04B\\User-Defined Variables\\ACV09A-Reading"(w259) -> ()  [unwired: 1 in, 1 out]
                n173 = shared-variable "FOFB-Controller\\Actuation Network\\PS-RA04B\\User-Defined Variables\\ACH07B-Reading"(w258) -> ()  [unwired: 1 in, 1 out]
                n174 = shared-variable "FOFB-Controller\\Actuation Network\\PS-RA04B\\User-Defined Variables\\ACV07B-Reading"(w257) -> ()  [unwired: 1 in, 1 out]
                n175 = shared-variable "FOFB-Controller\\Actuation Network\\PS-RA04B\\User-Defined Variables\\PS-RA04B-Status"(w265) -> ()  [unwired: 1 in, 1 out]
              }
              frame condition #4 {
                n176 = shared-variable "FOFB-Controller\\Actuation Network\\PS-RA05B\\User-Defined Variables\\ACH10-Reading"(w273) -> ()  [unwired: 1 in, 1 out]
                n177 = shared-variable "FOFB-Controller\\Actuation Network\\PS-RA05B\\User-Defined Variables\\RRA05B-Reading"(w272) -> ()  [unwired: 1 in, 1 out]
                n178 = shared-variable "FOFB-Controller\\Actuation Network\\PS-RA05B\\User-Defined Variables\\ALV10A-Reading"(w271) -> ()  [unwired: 1 in, 1 out]
                n179 = shared-variable "FOFB-Controller\\Actuation Network\\PS-RA05B\\User-Defined Variables\\ALV10B-Reading"(w270) -> ()  [unwired: 1 in, 1 out]
                n180 = shared-variable "FOFB-Controller\\Actuation Network\\PS-RA05B\\User-Defined Variables\\ACH11A-Reading"(w269) -> ()  [unwired: 1 in, 1 out]
                n181 = shared-variable "FOFB-Controller\\Actuation Network\\PS-RA05B\\User-Defined Variables\\ACV11A-Reading"(w268) -> ()  [unwired: 1 in, 1 out]
                n182 = shared-variable "FOFB-Controller\\Actuation Network\\PS-RA05B\\User-Defined Variables\\ACH09B-Reading"(w267) -> ()  [unwired: 1 in, 1 out]
                n183 = shared-variable "FOFB-Controller\\Actuation Network\\PS-RA05B\\User-Defined Variables\\ACV09B-Reading"(w266) -> ()  [unwired: 1 in, 1 out]
                n184 = shared-variable "FOFB-Controller\\Actuation Network\\PS-RA05B\\User-Defined Variables\\PS-RA05B-Status"(w274) -> ()  [unwired: 1 in, 1 out]
              }
              frame condition #5 {
                n185 = shared-variable "FOFB-Controller\\Actuation Network\\PS-RA06B\\User-Defined Variables\\ACH12-Reading"(w282) -> ()  [unwired: 1 in, 1 out]
                n186 = shared-variable "FOFB-Controller\\Actuation Network\\PS-RA06B\\User-Defined Variables\\RRA06B-Reading"(w281) -> ()  [unwired: 1 in, 1 out]
                n187 = shared-variable "FOFB-Controller\\Actuation Network\\PS-RA06B\\User-Defined Variables\\ALV12A-Reading"(w280) -> ()  [unwired: 1 in, 1 out]
                n188 = shared-variable "FOFB-Controller\\Actuation Network\\PS-RA06B\\User-Defined Variables\\ALV12B-Reading"(w279) -> ()  [unwired: 1 in, 1 out]
                n189 = shared-variable "FOFB-Controller\\Actuation Network\\PS-RA06B\\User-Defined Variables\\ACH01A-Reading"(w278) -> ()  [unwired: 1 in, 1 out]
                n190 = shared-variable "FOFB-Controller\\Actuation Network\\PS-RA06B\\User-Defined Variables\\ACV01A-Reading"(w277) -> ()  [unwired: 1 in, 1 out]
                n191 = shared-variable "FOFB-Controller\\Actuation Network\\PS-RA06B\\User-Defined Variables\\ACH11B-Reading"(w276) -> ()  [unwired: 1 in, 1 out]
                n192 = shared-variable "FOFB-Controller\\Actuation Network\\PS-RA06B\\User-Defined Variables\\ACV11B-Reading"(w275) -> ()  [unwired: 1 in, 1 out]
                n193 = shared-variable "FOFB-Controller\\Actuation Network\\PS-RA06B\\User-Defined Variables\\PS-RA06B-Status"(w283) -> ()  [unwired: 1 in, 1 out]
              }
            }
          }
        }
      }
    }
  }
